vi "analysis(SubVI).vi"(11 "본문":string) -> (3 "출력":T1)   [LabVIEW 2018]
panel:
  out "에러 출력 2":errorcluster caption="에러 출력"
  out "에러 출력":errorcluster
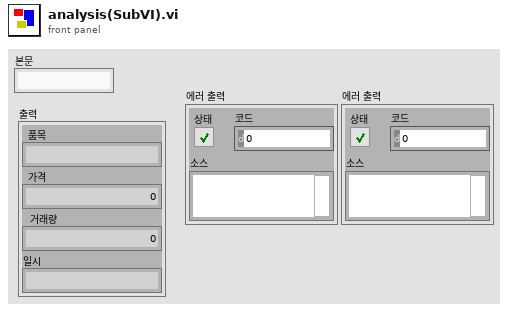
[diagram p1: front panel]
types:
  T1 = cluster{"품목":string, "가격":i32, "거래량":dbl, "일시":string}
  T2 = cluster{"본문":string, i32, "기본값 1":dbl, "본문":string}
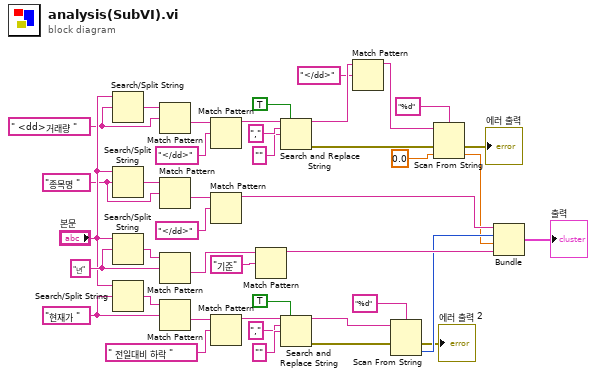
[diagram p0: block diagram]
diagram:
  w26 = "년" ("정규식")
  w17 = "종목명 " ("검색 문자열/문자 (-)")
  w7 = " <dd>거래량 " ("정규식")
  w13 = "현재가 " ("정규식")
  n1 = Search/Split String(string="본문", search string/char (-)=w7) -> (match + rest of string=w8:string)  [unwired: 1 in, 2 out]
  n2 = Search/Split String(string="본문", search string/char (-)=w17) -> (match + rest of string=w15:string)  [unwired: 1 in, 2 out]
  n3 = Search/Split String(string="본문", search string/char (-)=w26) -> (match + rest of string=w27:string)  [unwired: 1 in, 2 out]
  n4 = Search/Split String(string="본문", search string/char (-)=w13) -> (match + rest of string=w14:string)  [unwired: 1 in, 2 out]
  n5 = Match Pattern(string=w8, regular expression=w7) -> (after substring=w9:string)  [unwired: 1 in, 3 out]
  n6 = Match Pattern(string=w15, regular expression=w17) -> (after substring=w16:string)  [unwired: 1 in, 3 out]
  n7 = Match Pattern(string=w27, regular expression=w26) -> (after substring=w29:string)  [unwired: 1 in, 3 out]
  n8 = Match Pattern(string=w14, regular expression=w13) -> (after substring=w12:string)  [unwired: 1 in, 3 out]
  n9 = Match Pattern(string=w9, regular expression="</dd>" ("정규식")) -> (before substring=w38:string)  [unwired: 1 in, 3 out]
  n10 = Match Pattern(string=w16, regular expression="</dd>" ("정규식")) -> (before substring=w19:string)  [unwired: 1 in, 3 out]
  n11 = Match Pattern(string=w12, regular expression=" 전일대비 하락 " ("정규식")) -> (before substring=w33:string)  [unwired: 1 in, 3 out]
  n12 = Match Pattern(string=w29, regular expression="기준" ("정규식")) -> (before substring=w40:string)  [unwired: 1 in, 3 out]
  n13 = Search and Replace String(replace all?=TRUE ("모두 대체? (거짓)"), input string=w38, search string="," ("검색 문자열"), replace string="" ("대체 문자열(\"\")")) -> (result string=w39:string, error out=w1:errorcluster)  [unwired: 4 in, 2 out]
  n14 = Search and Replace String(replace all?=TRUE ("모두 대체? (거짓)"), input string=w33, search string="," ("검색 문자열"), replace string="" ("대체 문자열(\"\")")) -> (result string=w34:string, error out=w2:errorcluster)  [unwired: 4 in, 2 out]
  n15 = Match Pattern(string=w39, regular expression="</dd>" ("정규식")) -> (before substring=w21:string)  [unwired: 1 in, 3 out]
  n16 = Scan From String(format string="%d" ("포맷 문자열"), input string=w34, error in=w2) -> (error out=→"에러 출력 2":errorcluster, output 1=w6:i32)  [unwired: 2 in, 2 out]
  n17 = Scan From String(format string="%d" ("포맷 문자열"), input string=w21, error in=w1, default 1=0.0 ("기본값 1")) -> (error out=→"에러 출력":errorcluster, output 1=w5:dbl)  [unwired: 1 in, 2 out]
  n18 = Bundle("본문"=w19, w6, "기본값 1"=w5, "본문"=w40) -> (→"출력":T2)  [unwired: 1 in]
